vi "ReadFromFile(SubVI).vi"(2 "filter type":T1, 3 "Horni Mezni Frekvence (Hz)":dbl=0.45000000000000007 format="%0.2f", 4 "Dolni Mezni Frekvence (Hz)":dbl=0.12500000000000006 format="%0.4f", 5 "Sampling Freq":dbl) -> (0 "Amplitudove Spektrum":cluster{"f0":dbl, "df":dbl, "magnitude":dbl[]}, 1 "Waveform Graf":waveform(dbl))   [LabVIEW 2025]
uses:
  <vilib>/Analysis/3filter.llb/Filter Passband Type.ctl
  <vilib>/Analysis/4window.llb/windowTd.ctl
  <vilib>/Utility/file.llb/Read Delimited Spreadsheet (DBL).vi
  <vilib>/Analysis/3filter.llb/Butterworth Filter (DBL).vi
  <vilib>/measure/maspectr.llb/FFT Spectrum (Mag-Phase) for 1 Chan.vi
  <vilib>/measure/NI_MAPro.lvlib
  <vilib>/Analysis/NI_AALBase.lvlib
  <vilib>/Analysis/NI_AALPro.lvlib
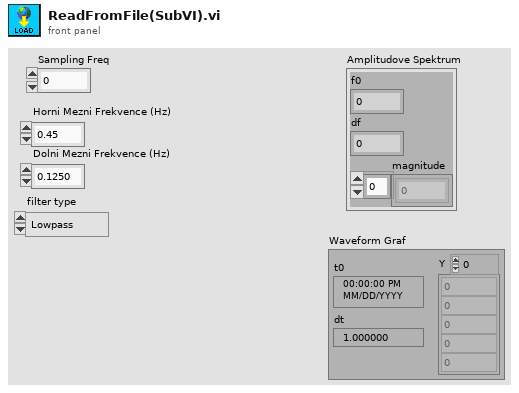
[diagram p1: front panel]
types:
  T1 = typedef "NI_AALBase.lvlib/Filter Passband Type.ctl" = enum32{"Lowpass", "Highpass", "Bandpass", "Bandstop"}
  T2 = typedef "NI_AALPro.lvlib/windowTd.ctl" = u32
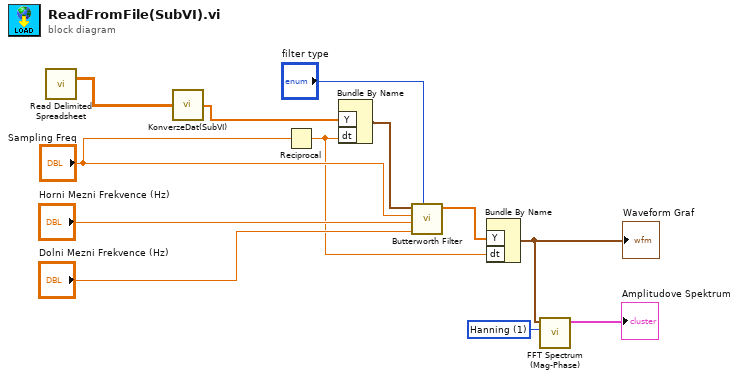
[diagram p0: block diagram]
diagram:
  w12 = T2 1 items=["Rectangle"=0, "Hanning"=1, "Hamming"=2, "Blackman-Harris"=3, "Exact Blackman"=4, "Blackman"=5, "Flat Top"=6, "4 Term B-Harris "=7, "7 Term B-Harris"=8, "Low Sidelobe"=9, "Blackman Nuttall"=11, "Triangle"=30, "Bartlett-Hanning"=31, "Bohman"=32, "Parzen"=33, "Welch"=34, "Kaiser"=60, "Dolph-Chebyshev"=61, "Gaussian"=62] ("window")
  n1 = call-poly <vilib>:"Read Delimited Spreadsheet.vi"() -> ("all rows"=w2:dbl[][])  [unwired: 10 in, 5 out]
  n2 = call "KonverzeDat(SubVI).vi"("Vstupni OpenSignals .txt export"=w2) -> ("Data ve spravnem formatu"=w1:dbl[])
  n3 = Reciprocal(x="Sampling Freq") -> (1/x=w4:dbl)
  n4 = Bundle By Name("Y"=w1, "dt"=w4) -> (w9:waveform(dbl))  [unwired: 1 in]
  n5 = call-poly <vilib>:"Butterworth Filter.vi"("filter type"="filter type", "low cutoff freq: fl"="Dolni Mezni Frekvence (Hz)", "high cutoff freq: fh"="Horni Mezni Frekvence (Hz)", "sampling freq: fs"="Sampling Freq", "X"=w9) -> ("Filtered X"=w10:dbl[])  [unwired: 3 in, 1 out]
  n6 = Bundle By Name("Y"=w10, "dt"=w4) -> (w11:waveform(dbl))  [unwired: 1 in]
  "Waveform Graf" <- w11
  n7 = call-poly <vilib>:"FFT Spectrum (Mag-Phase).vi"("window"=w12, "time signal"=w11) -> ("magnitude"=→"Amplitudove Spektrum":cluster{"f0":dbl, "df":dbl, "magnitude":dbl[]})  [unwired: 5 in, 4 out]
